vi "Point Data Updated.vi"(8 "error in":errorcluster, 9 "Data":variant, 10 "Point Ident":string, 11 "Sample PWM Tacho Fans in":refnum<class "Sample PWM Tacho Fans.lvclass">) -> (0 "error out":errorcluster, 3 "Sample PWM Tacho Fans out":refnum<class "Sample PWM Tacho Fans.lvclass">)   [LabVIEW 2023, in "Sample PWM Tacho Fans.lvlib" / "Sample PWM Tacho Fans.lvclass"]
doc: "Use this VI to update Point Data for repeatedly self calling Do.VI's"
uses:
  Sample PWM Tacho Fans.lvclass
  Sample PWM Tacho Fans.lvclass/Sample PWM Tacho Fans.ctl
  <vilib>/Utility/error.llb/Error Cluster From Error Code.vi
  <vilib>/ErrorRing/Error Ring.xnode
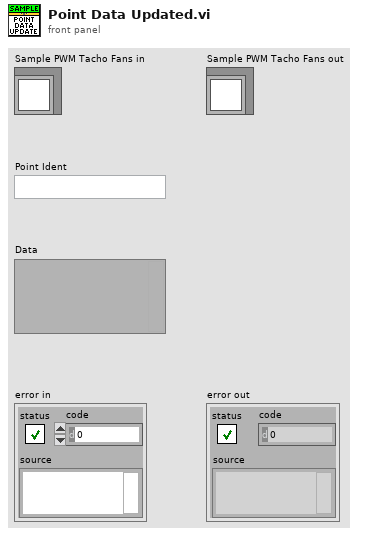
[diagram p1: front panel]
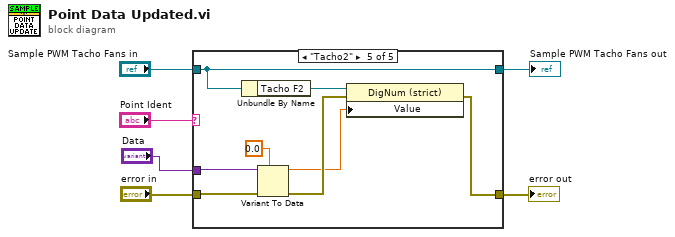
[diagram p0: block diagram]
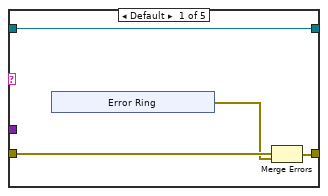
[diagram p2: hidden frame]
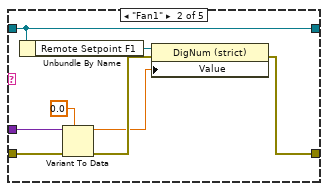
[diagram p3: hidden frame]
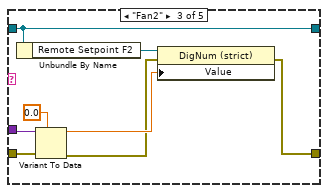
[diagram p4: hidden frame]
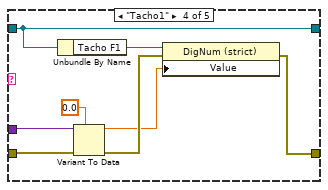
[diagram p5: hidden frame]
diagram:
  n1 = case shown="\"Tacho2\"" "Point Ident" {
    tunnel: "Sample PWM Tacho Fans in" -> [w10 w23 w31 w35 w43]
    tunnel: [w10 w23 w31 w35 w43] -> w5
    tunnel: [w9 w21 w24 w32 w40] -> w3
    tunnel: "error in" -> [w8 w20 w29 w33 w41]
    tunnel: "Data" -> [_ w18 w28 w34 w42]
    frame Default {
      n2 = xnode "Error Ring"() -> ("error out"=w7:errorcluster)
      n3 = Merge Errors(w8, w7) -> (w9:errorcluster)
    }
    frame "Fan1" {
      n4 = Unbundle By Name(w23) -> ("Remote Setpoint F1"=w22:refnum<vi>)
      n5 = Variant To Data(error in=w20, type=0.0, Variant=w18) -> (data=w16:dbl, error out=w19:errorcluster)
      n6 = property class="DigNum (strict)"(reference=w22, error in=w19, "Value"=w16) -> (error out=w21:errorcluster)  [unwired: 1 out]
    }
    frame "Fan2" {
      n7 = Unbundle By Name(w31) -> ("Remote Setpoint F2"=w30:refnum<vi>)
      n8 = Variant To Data(error in=w29, type=0.0, Variant=w28) -> (data=w26:dbl, error out=w25:errorcluster)
      n9 = property class="DigNum (strict)"(reference=w30, error in=w25, "Value"=w26) -> (error out=w24:errorcluster)  [unwired: 1 out]
    }
    frame "Tacho1" {
      n10 = Unbundle By Name(w35) -> ("Tacho F1"=w39:refnum<vi>)
      n11 = Variant To Data(error in=w33, type=0.0, Variant=w34) -> (data=w36:dbl, error out=w38:errorcluster)
      n12 = property class="DigNum (strict)"(reference=w39, error in=w38, "Value"=w36) -> (error out=w32:errorcluster)  [unwired: 1 out]
    }
    frame "Tacho2" {
      n13 = Unbundle By Name(w43) -> ("Tacho F2"=w47:refnum<vi>)
      n14 = Variant To Data(error in=w41, type=0.0, Variant=w42) -> (data=w44:dbl, error out=w46:errorcluster)
      n15 = property class="DigNum (strict)"(reference=w47, error in=w46, "Value"=w44) -> (error out=w40:errorcluster)  [unwired: 1 out]
    }
  }
  "error out" <- w3
  "Sample PWM Tacho Fans out" <- w5
